vi "QueryData.vi"(8 "error in (no error)":errorcluster, 10 "Query?":bool, 11 "4118 in":refnum<class "4118.lvclass">) -> (0 "error out":errorcluster, 3 "4118 out":refnum<class "4118.lvclass">)   [LabVIEW 2024, in "4118 Actor.lvlib" / "4118.lvclass"]
uses:
  4118.lvclass
  4118.lvclass/4118.ctl
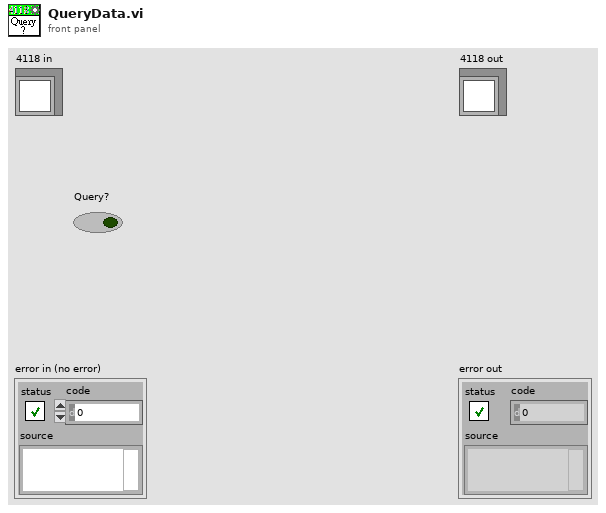
[diagram p1: front panel]
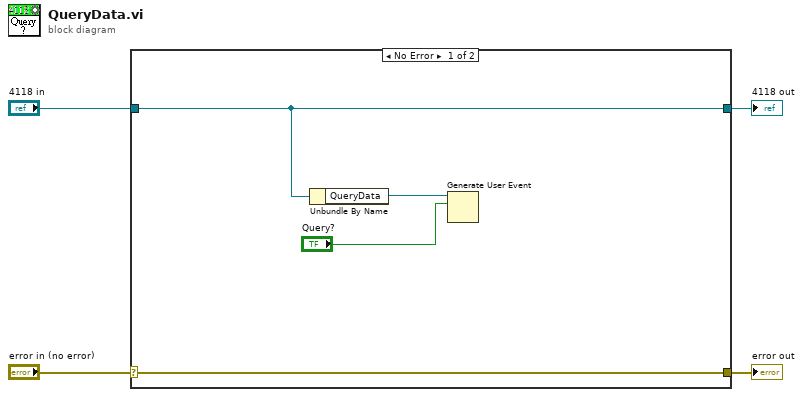
[diagram p0: block diagram]
diagram:
  n1 = case shown="No Error" "error in (no error)" {
    selector: "error in (no error)" -> [w8 w10]
    tunnel: [w8 w10] -> w3
    tunnel: [w7 w9] -> w1
    tunnel: "4118 in" -> [w7 w9]
    frame No Error {
      n2 = Unbundle By Name(w7) -> ("QueryData"=w6:refnum<user-event>)
      n3 = Generate User Event(user event=w6, event data cluster="Query?") -> ()  [unwired: 2 in, 2 out]
    }
    frame Error {
    }
  }
  "error out" <- w3
  "4118 out" <- w1
